vi "LV SciSDK TOF SPECTRUM.vi"(7 "TOF Spectrum Handle In":cluster{"TOF Path":string, "TOF Name":string}, 9 "Board Handle In":T1, 11 "error in (no error)":errorcluster) -> (4 "NI Error Code":i32, 6 "TOF Spectrum Buffer Out":T2, 8 "TOF Spectrum Handle Out":cluster{"TOF Path":string, "TOF Name":string}, 10 "Board Handle Out":T1, 15 "error out":errorcluster)   [LabVIEW 2021, in "SciSDK_Labview.lvlib"]
uses:
  SciSDK_Labview.lvlib
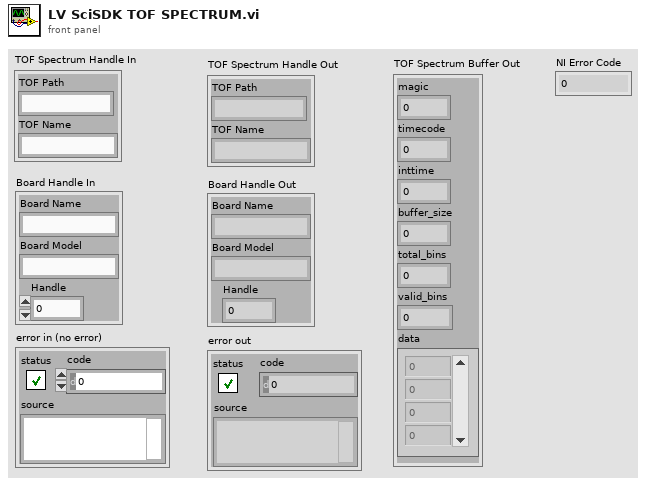
[diagram p1: front panel]
types:
  T1 = cluster{"Board Name":string, "Board Model":string, "Handle":u64}
  T2 = cluster{"magic":u32, "timecode":u32, "inttime":u32, "buffer_size":u32, "total_bins":u32, "valid_bins":u32, "data":i32[]}
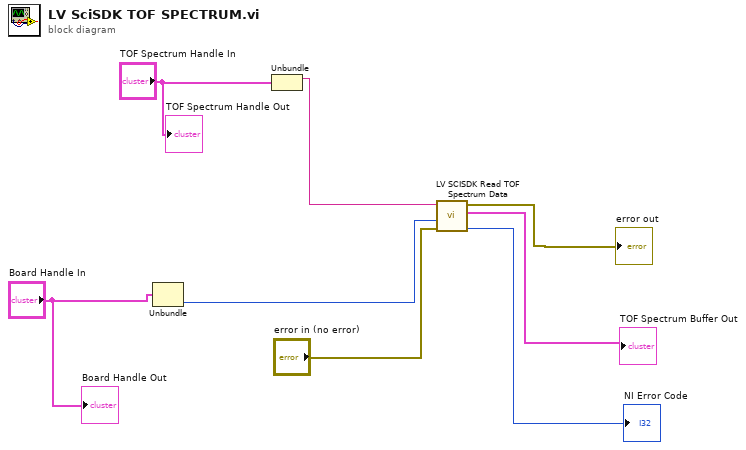
[diagram p0: block diagram]
diagram:
  n1 = Unbundle("Board Handle In") -> ("Handle"=w1:u64)  [unwired: 2 out]
  n2 = Unbundle("TOF Spectrum Handle In") -> ("TOF Path"=w3:string)  [unwired: 1 out]
  n3 = call "LV SCISDK Read TOF Spectrum Data.vi"("Path"=w3, "handle"=w1, "error in (no error)"="error in (no error)") -> ("error out"=→"error out":errorcluster, "buffer out"=→"TOF Spectrum Buffer Out":T2, "function return"=→"NI Error Code":i32)  [unwired: 4 in, 1 out]
  "TOF Spectrum Handle Out" <- "TOF Spectrum Handle In"
  "Board Handle Out" <- "Board Handle In"
